vi "serial port init.vi"(8 "错误输入（无错误）":errorcluster, 10 "海马(1)":bool, 11 "VISA引用句柄输入":refnum<visa-resource-name>="COM1") -> (0 "错误输出":errorcluster, 3 "VISA引用句柄输出":refnum<visa-resource-name>)   [LabVIEW 2013]
uses:
  C:/Program Files/National Instruments/LabVIEW 2013/examples/Instrument IO/Serial/support/Serial - Settings.ctl
  <vilib>/Instr/_visa.llb/VISA Flush IO Buffer Mask.ctl
  <vilib>/Instr/_visa.llb/VISA Configure Serial Port (Instr).vi
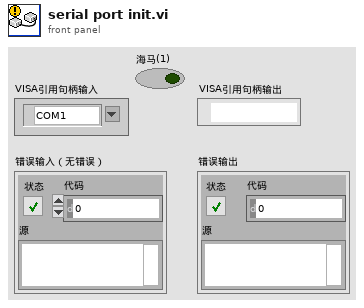
[diagram p1: front panel]
types:
  T1 = typedef "Serial - Settings.ctl" = cluster{"波特率":u32, "数据比特":u16, "奇偶":enum16{"None", "Odd", "Even", "Mark", "Space"}, "停止位":u16, "流控制":u16}
  T2 = typedef "VISA Flush IO Buffer Mask.ctl" = u16
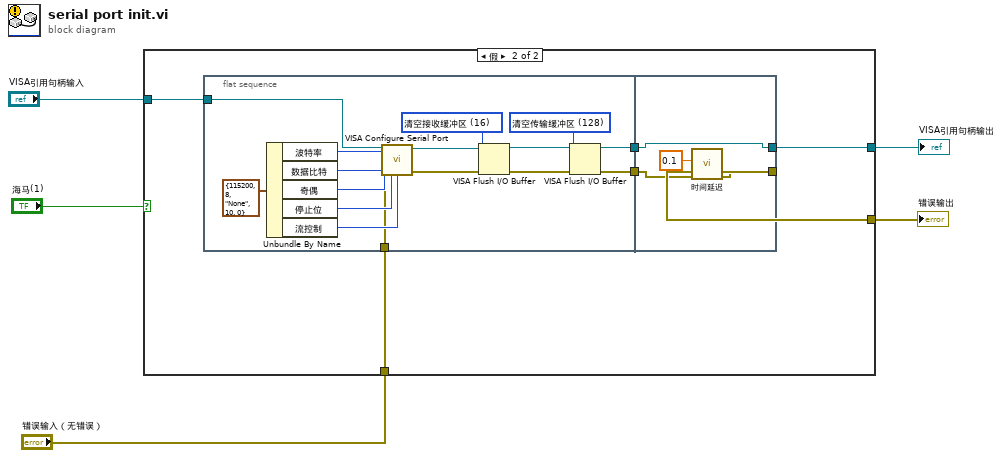
[diagram p0: block diagram]
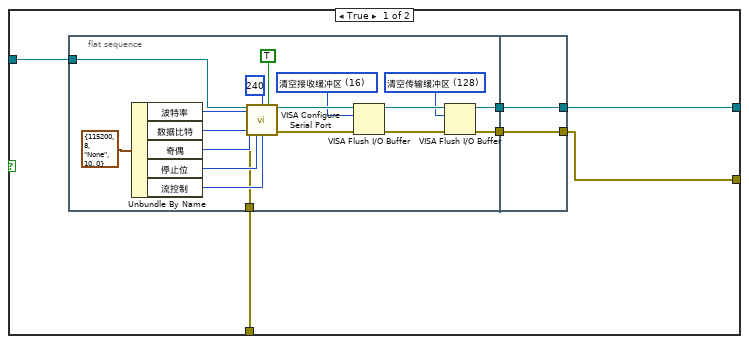
[diagram p2: hidden frame]
diagram:
  n1 = case shown="假" "海马(1)" {
    tunnel: [w9 w36] -> w5
    tunnel: [w8 w35] -> w4
    tunnel: "错误输入（无错误）" -> [w7 w34]
    tunnel: "VISA引用句柄输入" -> [w6 w33]
    frame True {
      n2 = flat-sequence {
        tunnel: w7 -> [w23]
        tunnel: [w17] -> w11
        tunnel: [w16] -> w10
        tunnel: w6 -> [w20]
        tunnel: [w30] -> w9
        tunnel: [w31] -> w8
        tunnel: w11 -> [w31]
        tunnel: w10 -> [w30]
        frame #0 {
          w12 = T2 128 items=["清空接收缓冲区"=16, "向设备写入传输缓冲区"=32, "清空接收缓冲区（无I/O）"=64, "清空传输缓冲区"=128] ("Mask")
          w13 = T2 16 items=["清空接收缓冲区"=16, "向设备写入传输缓冲区"=32, "清空接收缓冲区（无I/O）"=64, "清空传输缓冲区"=128] ("Mask")
          n3 = Unbundle By Name(T1 {"波特率"=115200, "数据比特"=8, "奇偶"=enum."None", "停止位"=10, "流控制"=0} ("串口设置")) -> ("波特率"=w26:u32, "数据比特"=w27:u16, "奇偶"=w28:enum16{"None", "Odd", "Even", "Mark", "Space"}, "停止位"=w29:u16, "流控制"=w24:u16)
          n4 = call-poly "VISA Configure Serial Port"("VISA resource name"=w20, "termination char\n(0xA = '\\n' = LF)"=u8 240 ("termination char\n(0xA = '\\n' = LF)"), "Enable Termination\nChar (T)"=TRUE ("Enable Termination\nChar (T)"), "baud rate (9600)"=w26, "data bits (8)"=w27, "parity (0:none)"=w28, "error in (no error)"=w23, "stop bits (10: 1 bit)"=w29, "flow control (0:none)"=w24) -> ("VISA resource name out"=w14:refnum<visa-resource-name>, "error out"=w15:errorcluster)  [unwired: 1 in, 4 out]
          n5 = VISA Flush I/O Buffer(VISA resource name=w14, mask (16)=w13, error in (no error)=w15) -> (VISA resource name out=w18:refnum<visa-resource-name>, error out=w19:errorcluster)
          n6 = VISA Flush I/O Buffer(VISA resource name=w18, mask (16)=w12, error in (no error)=w19) -> (VISA resource name out=w17:refnum<visa-resource-name>, error out=w16:errorcluster)
        }
        frame #1 {
        }
      }
    }
    frame False {
      n7 = flat-sequence {
        tunnel: w34 -> [w47]
        tunnel: [w40] -> w37
        tunnel: w33 -> [w44]
        tunnel: [w39] -> w32
        tunnel: [w54] -> w36
        tunnel: [w55] -> w35
        tunnel: w37 -> [w55]
        tunnel: w32 -> [w56]
        frame #0 {
          w38 = T2 128 items=["清空接收缓冲区"=16, "向设备写入传输缓冲区"=32, "清空接收缓冲区（无I/O）"=64, "清空传输缓冲区"=128] ("Mask")
          w43 = T2 16 items=["清空接收缓冲区"=16, "向设备写入传输缓冲区"=32, "清空接收缓冲区（无I/O）"=64, "清空传输缓冲区"=128] ("Mask")
          n8 = Unbundle By Name(T1 {"波特率"=115200, "数据比特"=8, "奇偶"=enum."None", "停止位"=10, "流控制"=0} ("串口设置")) -> ("波特率"=w50:u32, "数据比特"=w51:u16, "奇偶"=w52:enum16{"None", "Odd", "Even", "Mark", "Space"}, "停止位"=w53:u16, "流控制"=w48:u16)
          n9 = call-poly "VISA Configure Serial Port"("VISA resource name"=w44, "baud rate (9600)"=w50, "data bits (8)"=w51, "parity (0:none)"=w52, "error in (no error)"=w47, "stop bits (10: 1 bit)"=w53, "flow control (0:none)"=w48) -> ("VISA resource name out"=w45:refnum<visa-resource-name>, "error out"=w46:errorcluster)  [unwired: 3 in, 4 out]
          n10 = VISA Flush I/O Buffer(VISA resource name=w45, mask (16)=w43, error in (no error)=w46) -> (VISA resource name out=w41:refnum<visa-resource-name>, error out=w42:errorcluster)
          n11 = VISA Flush I/O Buffer(VISA resource name=w41, mask (16)=w38, error in (no error)=w42) -> (VISA resource name out=w40:refnum<visa-resource-name>, error out=w39:errorcluster)
        }
        frame #1 {
          n12 = call "时间延迟"("error in (no error)"=w56, "Delay Time (s)"=0.1) -> ("error out"=w54:errorcluster)  [unwired: 9 in]
        }
      }
    }
  }
  "错误输出" <- w5
  "VISA引用句柄输出" <- w4
